vi "325-Configure Instrument.vi"(0 "VISA resource name":refnum<visa-resource-name>, 5 "Keypad Lock (F: Off)":bool, 7 "Lock Code (123)":dbl=123.0, 9 "Remote Interface Mode (0:Local)":u16(ring) items=["Local", "Remote", "Remote with local lockout"], 11 "error in (no error)":errorcluster) -> (4 "VISA resource name out":refnum<visa-resource-name>, 15 "error out":errorcluster)   [LabVIEW 2019, in "Lake Shore 325.lvlib"]
doc: "This VI configures various instrument settings. Parameters configured are;\nRemote interface mode, and keypad lock out."
uses:
  Lake Shore 325.lvlib
  Instance           1 28Saved   Configure Instrument .vi
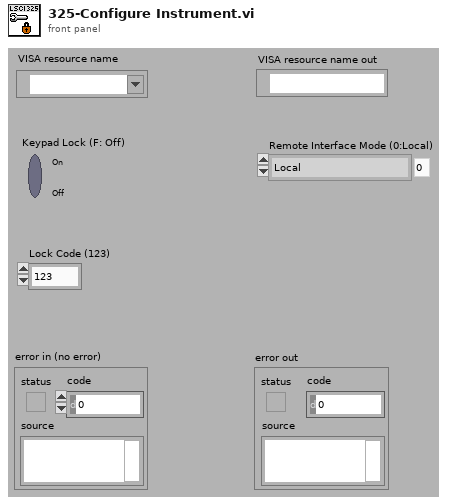
[diagram p1: front panel]
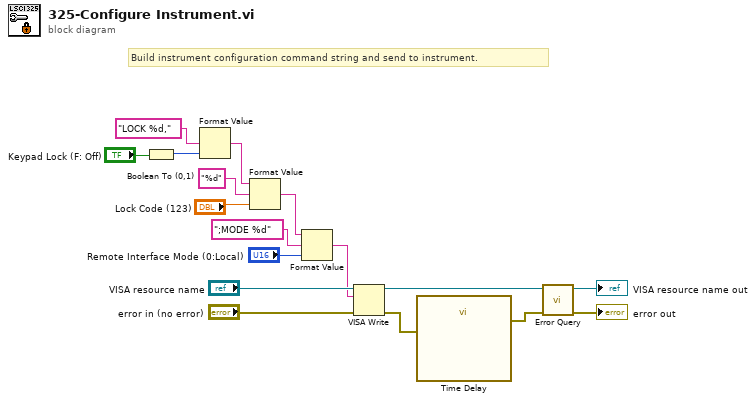
[diagram p0: block diagram]
diagram:
  # "Build instrument configuration command string and send to instrument."
  n1 = Boolean To (0,1)(Boolean="Keypad Lock (F: Off)") -> (0, 1=w10:i16)
  n2 = Format Value(format string="LOCK %d,", value (0)=w10) -> (output string=w3:string)  [unwired: 1 in]
  n3 = Format Value(string ("")=w3, format string="%d", value (0)="Lock Code (123)") -> (output string=w7:string)
  n4 = Format Value(string ("")=w7, format string=";MODE %d", value (0)="Remote Interface Mode (0:Local)") -> (output string=w5:string)
  n5 = VISA Write(VISA resource name="VISA resource name", write buffer=w5, error in (no error)="error in (no error)") -> (VISA resource name out=w15:refnum<visa-resource-name>, error out=w2:errorcluster)  [unwired: 1 out]
  n6 = call "Time Delay"("error in (no error)"=w2) -> ("error out"=w1:errorcluster)  [unwired: 10 in]
  n7 = call "Error Query.vi"("error in (no error)"=w1, "VISA resource name"=w15) -> ("error out"=→"error out":errorcluster, "VISA resource name out"=→"VISA resource name out":refnum<visa-resource-name>)  [unwired: 7 in, 1 out]
